vi "timestring.vi"() -> (5 "时间字符串":string)   [LabVIEW 2016, in "server.lvlib" / "server.lvclass"]
uses:
  server.lvclass
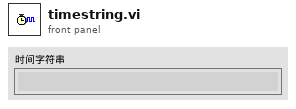
[diagram p1: front panel]
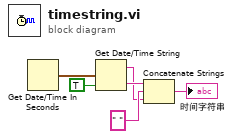
[diagram p0: block diagram]
diagram:
  n1 = Get Date/Time In Seconds() -> (seconds since 1Jan1904=w6:timestamp)
  n2 = Get Date/Time String(seconds (now)=w6, want seconds? (F)=TRUE ("需要秒？(F)")) -> (date string=w2:string, time string=w3:string)  [unwired: 1 in]
  n3 = Concatenate Strings(w3, " " ("字符串"), w2) -> (→"时间字符串":string)
